vi "Terminate.vi"(8 "error in (no error)":errorcluster, 10 "Message in":refnum<class "TerminateMessage.lvclass">, 11 "AOTF in":refnum<class "AOTF.lvclass">) -> (0 "error out":errorcluster, 3 "AOTF out":refnum<class "AOTF.lvclass">)   [LabVIEW 2012, in "AOTF.lvclass"]
doc: "This member function is called when the statemachine in the run.vi receives an 'terminate' command. It closes the RabbitMQ connection. \n\nOverride this member function in your derived class to release all previously acquired resources (but don't forget to call the parent method). If your component has subcomponents, they count as resources, and you have to release them by calling their own terminate functions."
uses:
  AOTF.lvclass
  <vilib>/Distrio/Murmex/TerminateMessage/TerminateMessage.lvclass
  <vilib>/Distrio/Murmex/Murmex/Murmex.lvclass
panel:
  # "This method is called when the TERMINATE\ntrigger is sent. \n\nOverride this method when your component needs to\nrespond to this trigger. \n\nCall parent for proper implementation"
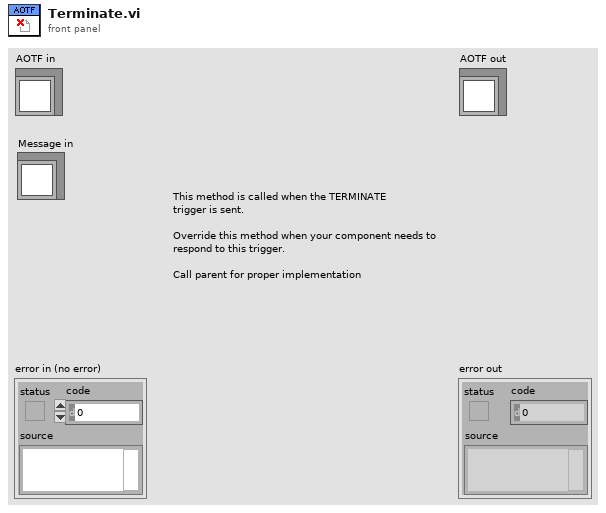
[diagram p1: front panel]
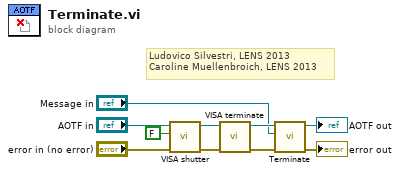
[diagram p0: block diagram]
diagram:
  # "Ludovico Silvestri, LENS 2013\nCaroline Muellenbroich, LENS 2013"
  n1 = call-dynamic "VISA shutter.vi"("error in (no error)"="error in (no error)", "button::shutter"=FALSE, "AOTF in"="AOTF in") -> ("error out"=w4:errorcluster, "AOTF out"=w5:refnum<class "AOTF.lvclass">)  [unwired: 7 in]
  n2 = call-dynamic "VISA terminate.vi"("error in (no error)"=w4, "AOTF in"=w5) -> ("error out"=w7:errorcluster, "AOTF out"=w8:refnum<class "AOTF.lvclass">)  [unwired: 8 in]
  n3 = call-parent "Terminate.vi"("error in (no error)"=w7, "Message in"="Message in", "Murmex in"=w8) -> ("error out"=→"error out":errorcluster, "Murmex out"=→"AOTF out":refnum<class "AOTF.lvclass">)  [unwired: 7 in]
